vi "Enhong PID Ramp.vi"() -> ()   [LabVIEW 2015]
uses:
  <vilib>/Instr/_visa.llb/VISA Configure Serial Port (Instr).vi
panel:
  out "Waveform Graph":dbl[](graph)
  out "New ramp":u32
  out "Numeric":i32
  out "New ramp":string
  out "hex integer string":string
  out "number 2":i32
  out "hrs":u32
  out "mins":u32
  in  "Ramp time (mins)":u32
  out "number":dbl
  out "concatenated string":string
  out "read buffer":string
  in  "Setpoint":dbl
  in  "stop":bool
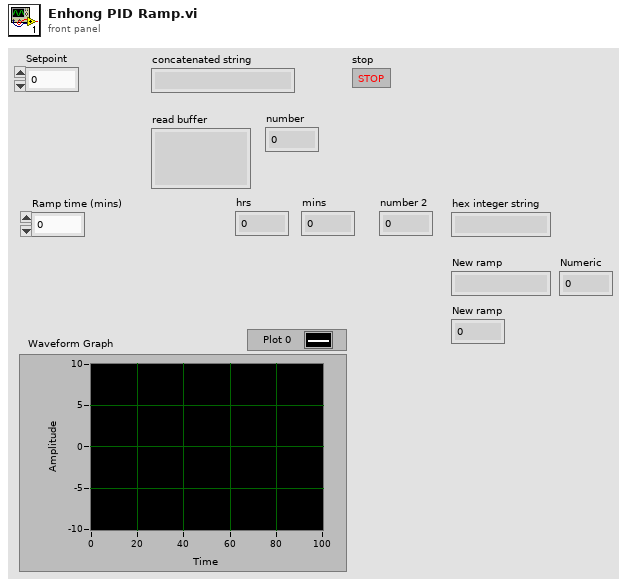
[diagram p1: front panel]
types:
  T1 = enum16{"Initialise ramp", "Default", "New Setpoint", "Ramp", "End Ramp"}
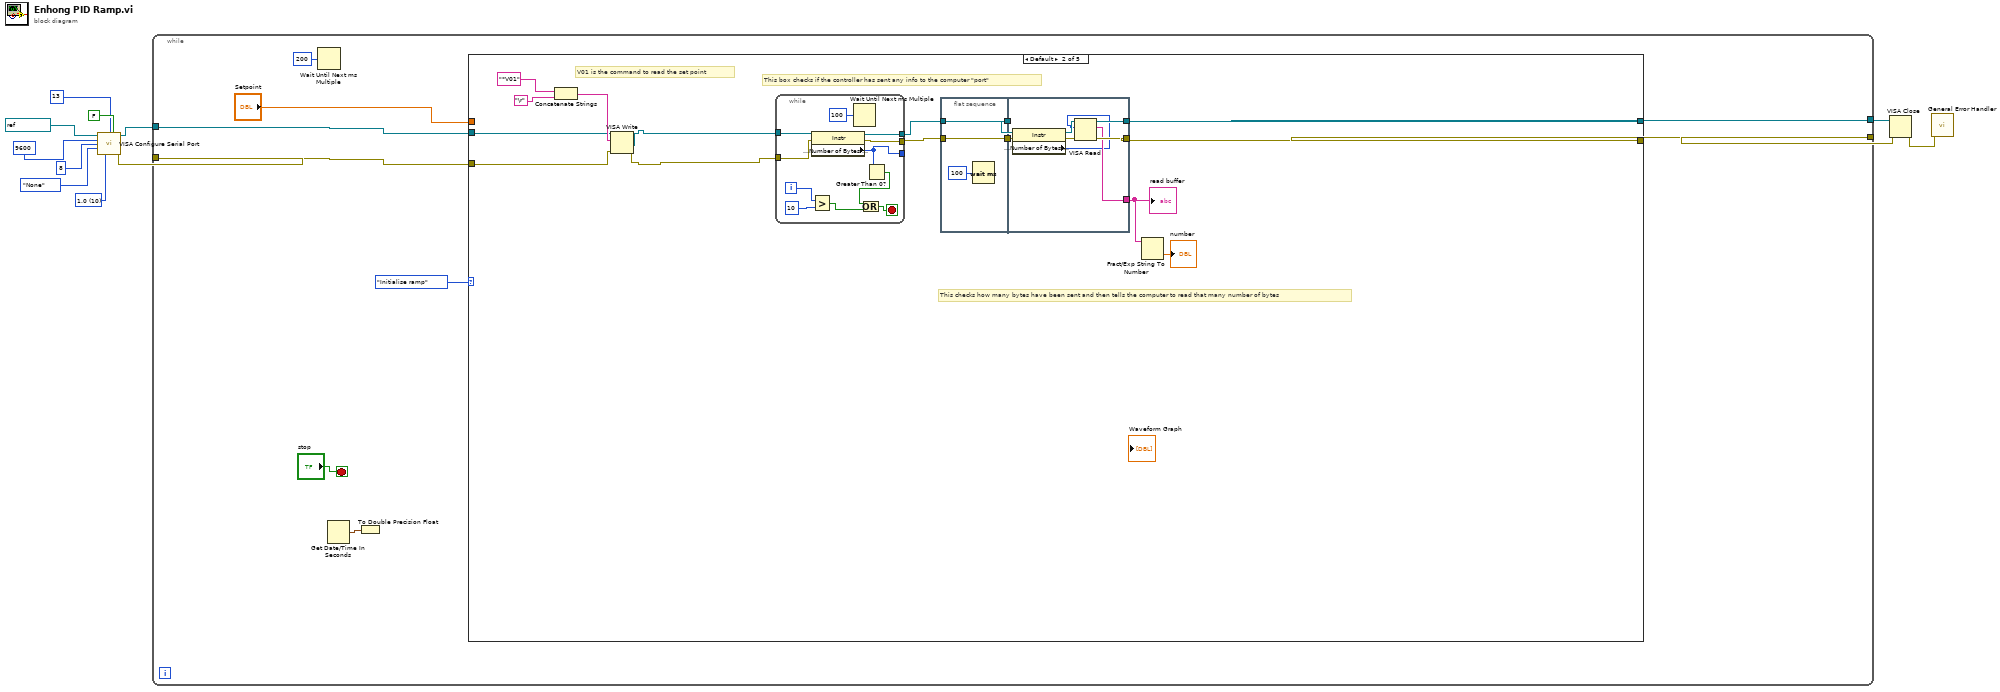
[diagram p0: block diagram]
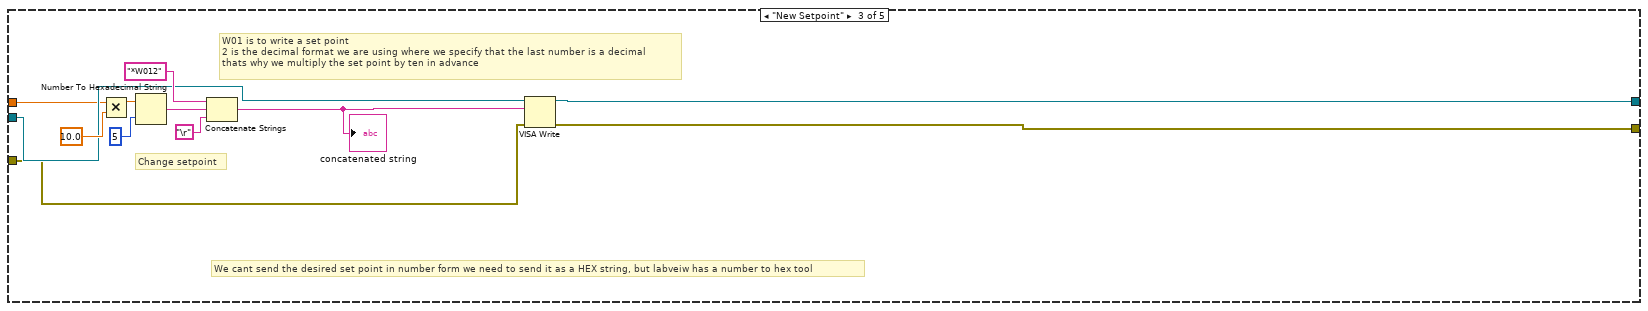
[diagram p3: hidden frame]
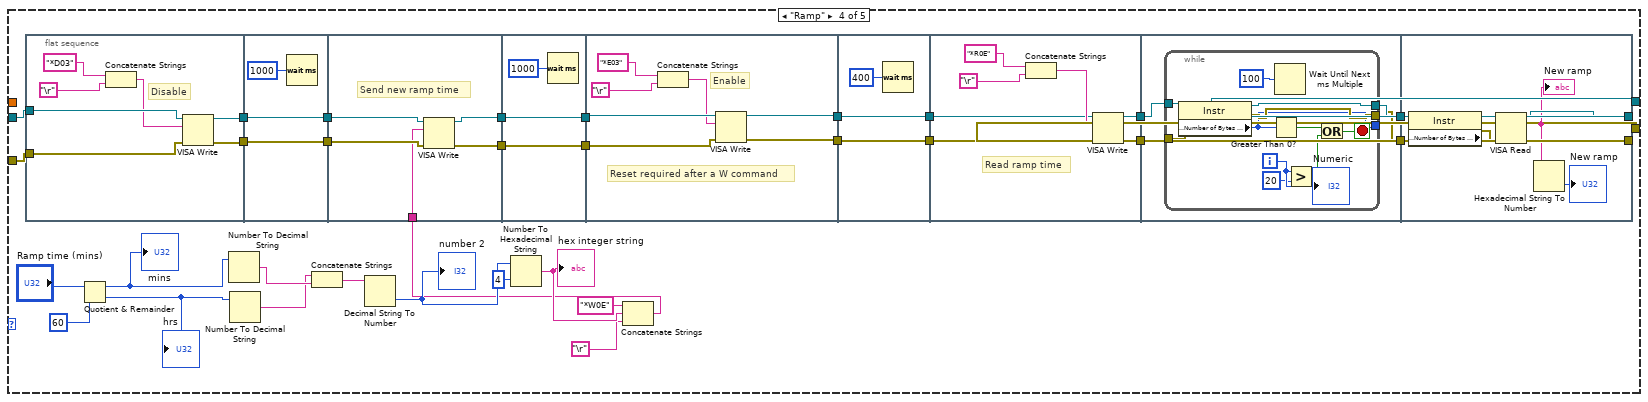
[diagram p4: hidden frame]
diagram:
  w3 = u16 10 items=["1.0"=10, "1.5"=15, "2.0"=20] ("stop bits (10: 1 bit)")
  n1 = call-poly "VISA Configure Serial Port"("VISA resource name"=refnum<visa-resource-name> "COM5", "termination char\n(0xA = '\\n' = LF)"=u8 13 ("termination char\n(0xA = '\\n' = LF)"), "Enable Termination\nChar (T)"=FALSE ("Enable Termination\nChar (T)"), "baud rate (9600)"=u32 9600, "data bits (8)"=u16 8, "parity (0:none)"=enum16{"None", "Odd", "Even", "Mark", "Space"}."None", "stop bits (10: 1 bit)"=w3) -> ("VISA resource name out"=w11:refnum<visa-resource-name>, "error out"=w10:errorcluster)  [unwired: 7 in]
  n2 = while {
    tunnel: [w17] -> w1
    tunnel: [w16] -> w12
    tunnel: w11 -> [w19]
    tunnel: w10 -> [w18]
    stop <- "stop" stop-if-true
    n3 = Wait Until Next ms Multiple(millisecond multiple=u32 200) -> ()  [unwired: 1 out]
    n4 = Get Date/Time In Seconds() -> (seconds since 1Jan1904=w14:timestamp)
    n5 = To Double Precision Float(number=w14) -> ()  [unwired: 1 out]
    n6 = case shown="Default" T1."Initialise ramp" {
      tunnel: w19 -> [w22 w27 w65 w95 w166]
      tunnel: w18 -> [w23 w26 w64 w94 w165]
      tunnel: [w22 w25 w63 w96 w166] -> w17
      tunnel: [w23 w24 w62 w97 w165] -> w16
      tunnel: "Setpoint" -> [_ _ w61 _ _]
      frame "Initialise ramp" {
      }
      frame Default {
        # "This checks how many bytes have been sent and then tells the computer to read that many number of bytes"
        # "This box checks if the controller has sent any info to the computer \"port\""
        # "V01 is the command to read the set point"
        n7 = Concatenate Strings("*V01" ("string"), "\r") -> (w36:string)
        n8 = VISA Write(VISA resource name=w27, write buffer=w36, error in (no error)=w26) -> (VISA resource name out=w32:refnum<visa-resource-name>, error out=w33:errorcluster)  [unwired: 1 out]
        n9 = while {
          tunnel: w32 -> [w57]
          tunnel: [w55] -> w31
          tunnel: [w54] -> w30
          tunnel: [w53] -> _
          tunnel: w33 -> [w50]
          i -> [w52]
          stop <- w59 stop-if-true
          n10 = Greater?(x=w52, y=10 ("x")) -> (0:w58:bool)
          n11 = property class="Instr"(reference=w57, error in=w50) -> (reference out=w55:refnum<visa-resource-name>, error out=w54:errorcluster, "Serial Settings:Number of Bytes at Serial Port"=w53:u32)
          n12 = Wait Until Next ms Multiple(millisecond multiple=u32 100) -> ()  [unwired: 1 out]
          n13 = Greater Than 0?(x=w53) -> (x > 0?=w56:bool)
          n14 = Or(x=w56, y=w58) -> (x .or. y?=w59:bool)
        }
        n15 = flat-sequence {
          tunnel: w31 -> [w41]
          tunnel: [w41] -> w38
          tunnel: w30 -> [w40]
          tunnel: [w40] -> w37
          tunnel: [w49] -> w25
          tunnel: [w48] -> w24
          tunnel: w38 -> [w46]
          tunnel: [w47] -> w29
          tunnel: w37 -> [w42]
          frame #0 {
            n16 = Wait (ms)(milliseconds to wait=u32 100) -> ()  [unwired: 1 out]
          }
          frame #1 {
            n17 = property class="Instr"(reference=w46, error in=w42) -> (reference out=w45:refnum<visa-resource-name>, error out=w44:errorcluster, "Serial Settings:Number of Bytes at Serial Port"=w43:u32)
            n18 = VISA Read(VISA resource name=w45, byte count=w43, error in (no error)=w44) -> (VISA resource name out=w49:refnum<visa-resource-name>, read buffer=w47:string, error out=w48:errorcluster)  [unwired: 1 out]
          }
        }
        n19 = Fract/Exp String To Number(string=w29) -> (number=→"number":dbl)  [unwired: 3 in, 1 out]
        "read buffer" <- w29
      }
      frame "New Setpoint" {
        # "We cant send the desired set point in number form we need to send it as a HEX string, but labveiw has a number to hex tool"
        # "W01 is to write a set point\n2 is the decimal format we are using where we specify that the last number is a decimal\nthats why we multiply the set point by ten in advance"
        # "Change setpoint"
        n20 = Multiply(x=w61, y=10.0) -> (x*y=w69:dbl)
        n21 = Number To Hexadecimal String(1:i16 5 ("width (-)"), 2:w69) -> (0:w67:string)
        n22 = Concatenate Strings("*W012" ("string"), w67, "\r") -> (w72:string)
        "concatenated string" <- w72
        n23 = VISA Write(VISA resource name=w65, write buffer=w72, error in (no error)=w64) -> (VISA resource name out=w63:refnum<visa-resource-name>, error out=w62:errorcluster)  [unwired: 1 out]
      }
      frame "Ramp" {
        n24 = flat-sequence {
          tunnel: w95 -> [w107]
          tunnel: w94 -> [w108]
          tunnel: [w109] -> w91
          tunnel: [w110] -> w82
          tunnel: [w114] -> w93
          tunnel: [w113] -> w92
          tunnel: w91 -> [w113]
          tunnel: w82 -> [w114]
          tunnel: w93 -> [w118]
          tunnel: w92 -> [w117]
          tunnel: [w120] -> w90
          tunnel: [w119] -> w87
          tunnel: w83 -> [w116]
          tunnel: w90 -> [w122]
          tunnel: [w122] -> w89
          tunnel: [w121] -> w88
          tunnel: w87 -> [w121]
          tunnel: w89 -> [w125]
          tunnel: w88 -> [w126]
          tunnel: [w127] -> w78
          tunnel: [w128] -> w76
          tunnel: w78 -> [w133]
          tunnel: [w133] -> w77
          tunnel: w76 -> [w132]
          tunnel: [w132] -> w75
          tunnel: [w136] -> w81
          tunnel: [w137] -> w80
          tunnel: w77 -> [w135]
          tunnel: w75 -> [w134]
          tunnel: w81 -> [w144]
          tunnel: w80 -> [w143]
          tunnel: [w142] -> w79
          tunnel: [w141] -> w74
          tunnel: [w164] -> w96
          tunnel: [w163] -> w97
          tunnel: w79 -> [w158]
          tunnel: w74 -> [w159]
          frame #0 {
            # "Disable"
            n25 = Concatenate Strings("*D03" ("write buffer"), "\r") -> (w106:string)
            n26 = VISA Write(VISA resource name=w107, write buffer=w106, error in (no error)=w108) -> (VISA resource name out=w110:refnum<visa-resource-name>, error out=w109:errorcluster)  [unwired: 1 out]
          }
          frame #1 {
            n27 = Wait (ms)(milliseconds to wait=u32 1000) -> ()  [unwired: 1 out]
          }
          frame #2 {
            # "Send new ramp time"
            n28 = VISA Write(VISA resource name=w118, write buffer=w116, error in (no error)=w117) -> (VISA resource name out=w120:refnum<visa-resource-name>, error out=w119:errorcluster)  [unwired: 1 out]
          }
          frame #3 {
            n29 = Wait (ms)(milliseconds to wait=u32 1000) -> ()  [unwired: 1 out]
          }
          frame #4 {
            # "Reset required after a W command"
            # "Enable"
            n30 = Concatenate Strings("*E03" ("write buffer"), "\r") -> (w124:string)
            n31 = VISA Write(VISA resource name=w125, write buffer=w124, error in (no error)=w126) -> (VISA resource name out=w128:refnum<visa-resource-name>, error out=w127:errorcluster)  [unwired: 1 out]
          }
          frame #5 {
            n32 = Wait (ms)(milliseconds to wait=u32 400) -> ()  [unwired: 1 out]
          }
          frame #6 {
            # "Read ramp time"
            n33 = Concatenate Strings("*R0E" ("write buffer"), "\r") -> (w138:string)
            n34 = VISA Write(VISA resource name=w134, write buffer=w138, error in (no error)=w135) -> (VISA resource name out=w137:refnum<visa-resource-name>, error out=w136:errorcluster)  [unwired: 1 out]
          }
          frame #7 {
            n35 = while {
              tunnel: w143 -> [w152]
              tunnel: [w150] -> w142
              tunnel: [w149] -> w141
              tunnel: [w148] -> _
              tunnel: w144 -> [w145]
              i -> [w147]
              stop <- w154 stop-if-true
              n36 = property class="Instr"(reference=w152, error in=w145) -> (reference out=w150:refnum<visa-resource-name>, error out=w149:errorcluster, "Serial Settings:Number of Bytes at Serial Port"=w148:u32)
              n37 = Greater Than 0?(x=w148) -> (x > 0?=w151:bool)
              n38 = Wait Until Next ms Multiple(millisecond multiple=u32 100) -> ()  [unwired: 1 out]
              n39 = Greater?(x=w147, y=20 ("x")) -> (0:w153:bool)
              n40 = Or(x=w151, y=w153) -> (x .or. y?=w154:bool)
              "Numeric" <- w147
            }
          }
          frame #8 {
            n41 = property class="Instr"(reference=w158, error in=w159) -> (reference out=w161:refnum<visa-resource-name>, error out=w160:errorcluster, "Serial Settings:Number of Bytes at Serial Port"=w162:u32)
            n42 = VISA Read(VISA resource name=w161, byte count=w162, error in (no error)=w160) -> (VISA resource name out=w164:refnum<visa-resource-name>, read buffer=w157:string, error out=w163:errorcluster)  [unwired: 1 out]
            "New ramp" <- w157
            n43 = Hexadecimal String To Number(string=w157) -> (number=→"New ramp":u32)  [unwired: 2 in, 1 out]
          }
        }
        n44 = Quotient & Remainder(x="Ramp time (mins)", y=u32 60) -> (x-y*floor(x/y)=w100:u32, floor(x/y)=w101:u32)
        "mins" <- w100
        "hrs" <- w101
        n45 = Number To Decimal String(number=w100) -> (decimal integer string=w103:string)  [unwired: 1 in]
        n46 = Number To Decimal String(number=w101) -> (decimal integer string=w102:string)  [unwired: 1 in]
        n47 = Concatenate Strings(w102, w103) -> (w104:string)
        n48 = Decimal String To Number(string=w104) -> (number=w105:i32)  [unwired: 2 in, 1 out]
        "number 2" <- w105
        n49 = Number To Hexadecimal String(1:i16 4 ("width (-)"), 2:w105) -> (0:w85:string)
        "hex integer string" <- w85
        n50 = Concatenate Strings("*W0E" ("string"), w85, "\r") -> (w83:string)
      }
      frame "End Ramp" {
      }
    }
  }
  n51 = VISA Close(VISA resource name=w1, error in (no error)=w12) -> (error out=w2:errorcluster)
  n52 = call <vilib>:"General Error Handler.vi"("error in (no error)"=w2) -> ()  [unwired: 10 in, 5 out]
